vi "Find Topology by Name.vi"(10 "Topology Name In":string, 11 "Topologies":T1[](array[typedef])) -> (2 "index":i32, 3 "Topology":T1)   [LabVIEW 2017, in "SLSC Switch.lvlib" / "SLSC Switch.lvclass"]
uses:
  SLSC Switch.lvclass
  Controls/Topology.ctl
  Controls/JSON.InitialState.ctl
  Controls/JSON.ChannelList.ctl
  Controls/JSON.ConnectionList.ctl
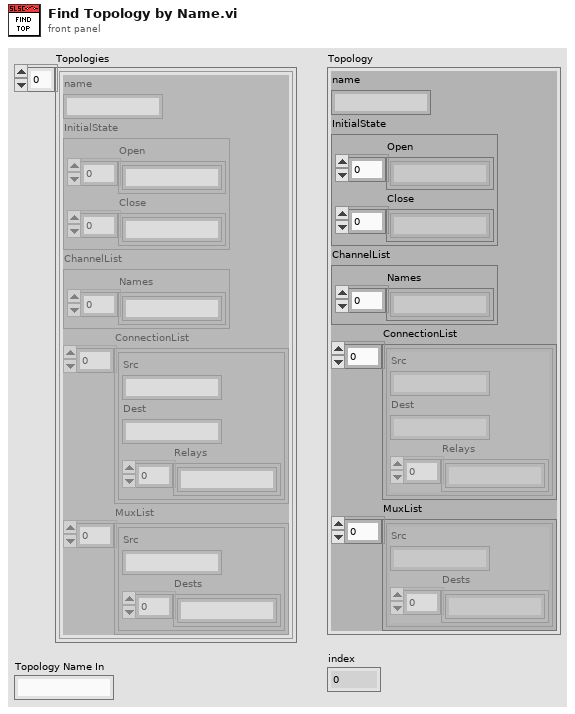
[diagram p1: front panel]
types:
  T1 = typedef "SLSC Switch.lvlib/SLSC Switch.lvclass/Topology.ctl" = cluster{"name":string, "InitialState":T2, "ChannelList":T3, "ConnectionList":T4[], "MuxList":cluster{"Src":string, "Dests":string[]}[]}
  T2 = typedef "SLSC Switch.lvlib/SLSC Switch.lvclass/JSON.InitialState.ctl" = cluster{"Open":string[], "Close":string[]}
  T3 = typedef "SLSC Switch.lvlib/SLSC Switch.lvclass/JSON.ChannelList.ctl" = cluster{"Names":string[]}
  T4 = typedef "SLSC Switch.lvlib/SLSC Switch.lvclass/JSON.ConnectionList.ctl" = cluster{"Src":string, "Dest":string, "Relays":string[]}
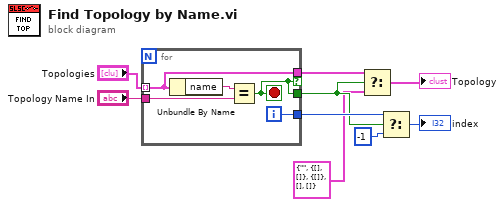
[diagram p0: block diagram]
diagram:
  n1 = for {
    tunnel: "Topologies" -> [w10] mode=indexing
    tunnel: "Topology Name In" -> [w14]
    tunnel: [w11] -> w4
    tunnel: [w13] -> w6
    tunnel: [w10] -> w3 if=w11
    i -> [w13]
    stop <- w11 stop-if-true
    n2 = Unbundle By Name(w10) -> ("name"=w12:string)
    n3 = Equal?(x=w12, y=w14) -> (x = y?=w11:bool)
  }
  n4 = Select(t=w3, s=w4, f=T1 {"name"="", "InitialState"={"Open"=[], "Close"=[]}, "ChannelList"={"Names"=[]}, "ConnectionList"=[], "MuxList"=[]}) -> (s? t:f=→"Topology":T1)
  n5 = Select(t=w6, s=w4, f=-1) -> (s? t:f=→"index":i32)
